vi "State Tracker Send Sample.vi"(8 "error in (no error)":errorcluster, 11 "RDS State Tracker in":refnum<class "RDS State Tracker.lvclass">) -> (0 "error out":errorcluster, 3 "RDS State Tracker out":refnum<class "RDS State Tracker.lvclass">)   [LabVIEW 2015, in "RDS State Tracker.lvlib" / "RDS State Tracker.lvclass"]
uses:
  RDS State Tracker.lvclass
  Libraries/RDS Child Messages/State Sample Message/State Sample Message.lvclass
  Libraries/RDS Framework/RDS Message ID.ctl
  RDS State Tracker.lvclass/RDS State Tracker.ctl
  Libraries/RDS Framework/RDS Message Class/RDS Message.lvclass/RDS Message.ctl
  Libraries/RDS Child Messages/State Sample Message/State Sample Message.lvclass/State Sample Message.ctl
  Actors/RDS Parent Actor/RDS Parent Actor/RDS Parent Actor.lvclass
  Libraries/RDS Framework/RDS Message Class/RDS Message.lvclass
  Libraries/RDS Child Messages/RDS Child Messages.lvlib
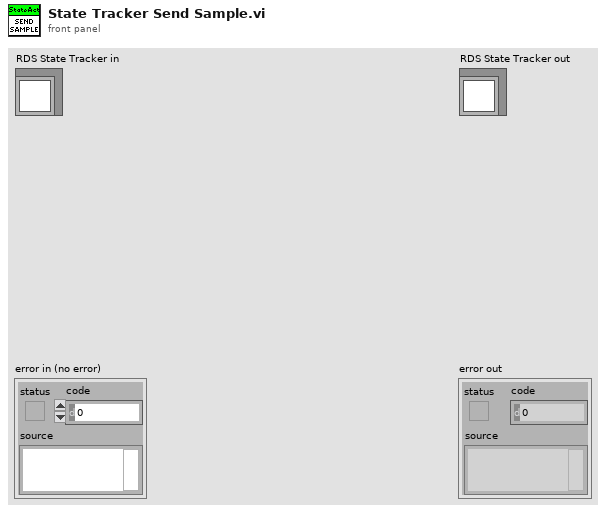
[diagram p1: front panel]
types:
  T1 = typedef "RDS Child Messages.lvlib/RDS Message ID.ctl" = enum16{"RDS Hello World", "String Message", "AIP_Status", "AIP_Command", "GPS_Data", "MCB_Command", "MCB_Status", "Compass_Data", "Depth_Data", "Battery_Data", "Contoller_State", "Set_Mag_Dev", "BTB_Shutdown", "State_Sample_Request", "State_Sample", "PID_Gains_Set", "Helm_Limiter_Set", "Helm_Heading_Command", "Helm_Steering_Command", "Helm_Status", "Controller_Message", "AIP_Set_Min_Depth", "Mission_Controller_State", "Mission_Upload", "Mission_Set_Op_and_Run", "Mission_Settings_Set"}
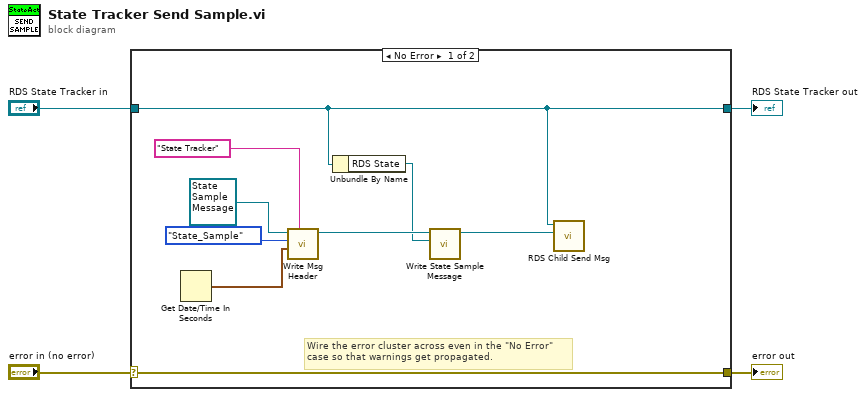
[diagram p0: block diagram]
diagram:
  n1 = case shown="No Error" "error in (no error)" {
    selector: "error in (no error)" -> [w13 w15]
    tunnel: [w13 w15] -> w3
    tunnel: [w5 w14] -> w1
    tunnel: "RDS State Tracker in" -> [w5 w14]
    frame No Error {
      # "Wire the error cluster across even in the \"No Error\"\ncase so that warnings get propagated."
      n2 = Get Date/Time In Seconds() -> (seconds since 1Jan1904=w9:timestamp)
      n3 = call "Write Msg Header.vi"("Sender Name"="State Tracker", "Time Stamp"=w9, "Msg ID"=RDS_Message_ID."State_Sample", "RDS Message in"=refnum<class "State Sample Message.lvclass"> refnum ("RDS Child Messages.lvlib:State Sample Message.lvclass")) -> ("RDS Message out"=w8:refnum<class "State Sample Message.lvclass">)  [unwired: 6 in, 1 out]
      n4 = Unbundle By Name(w5) -> ("RDS State"=w6:refnum<class "RDS State.lvclass">)
      n5 = call "Write State Sample Message.vi"("RDS State Tracker.lvlib:RDS State.lvclass"=w6, "State Sample Message in"=w8) -> ("State Sample Message out"=w7:refnum<class "State Sample Message.lvclass">)  [unwired: 8 in, 1 out]
      n6 = call "RDS Child Send Msg.vi"("RDS Message"=w7, "RDS Parent Actor in"=w5) -> ()  [unwired: 8 in, 2 out]
    }
    frame Error {
    }
  }
  "error out" <- w3
  "RDS State Tracker out" <- w1
